vi "getConfigNames.vi"(8 "error in (no error)":errorcluster, 11 "HWConfiguration in":refnum<class "HWConfigurations.lvclass">) -> (0 "error out":errorcluster, 2 "config_names":string[](array[string]), 3 "HWConfiguration out":refnum<class "HWConfigurations.lvclass">)   [LabVIEW 2009, in "Tools.lvlib" / "DatabaseHelpers.lvlib" / "HWConfigurations.lvclass"]
uses:
  HWConfigurations.lvclass
  HWConfigurations.lvclass/HWConfigurations.ctl
  OutputConfiguration/OutputConfiguration.lvclass
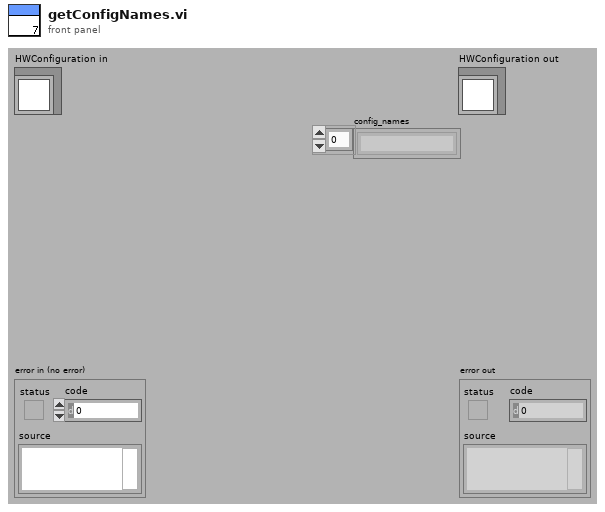
[diagram p1: front panel]
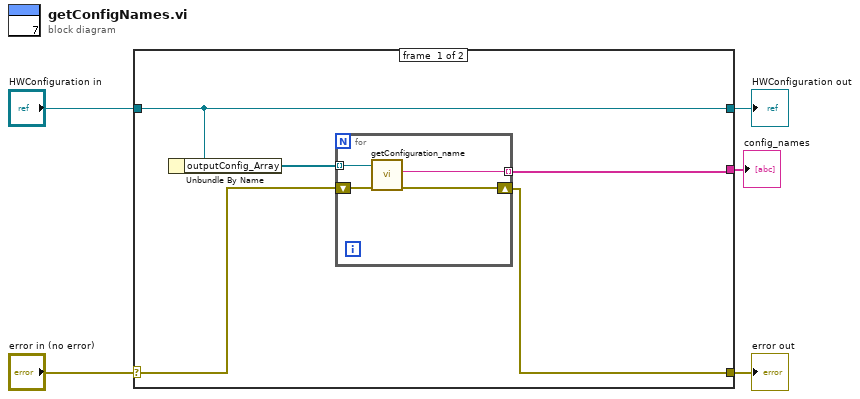
[diagram p0: block diagram]
diagram:
  n1 = case shown="No Error" "error in (no error)" {
    selector: "error in (no error)" -> [w7 w16]
    tunnel: [w6 w16] -> w4
    tunnel: [w10 w15] -> w2
    tunnel: "HWConfiguration in" -> [w10 w15]
    tunnel: [w8 _] -> w1
    frame #0 {
      n2 = Unbundle By Name(w10) -> ("outputConfig_Array"=w9:refnum<class "OutputConfiguration.lvclass">[])
      n3 = for {
        tunnel: w9 -> [w14] mode=indexing
        tunnel: [w13] -> w8 mode=indexing
        shift-right: [w11] -> w6
        shift-left: w7 -> [w12]
        n4 = call-dynamic "getConfiguration_name.vi"("error in (no error)"=w12, "OutputConfiguration.lvclass in"=w14) -> ("error out"=w11:errorcluster, "configuration_name"=w13:string)  [unwired: 7 in, 1 out]
      }
    }
    frame #1 {
    }
  }
  "error out" <- w4
  "HWConfiguration out" <- w2
  "config_names" <- w1
